vi "getHelpQuestionmark.vi"(8 "error in (no error)":errorcluster, 11 "TEI9150 in":refnum<class "TEI9150.lvclass">) -> (0 "error out":errorcluster, 2 "Items and Unit Numbers":string, 3 "TEI9150 out":refnum<class "TEI9150.lvclass">)   [LabVIEW 2015, in "TEI9150.lvclass"]
uses:
  TEI9150.lvclass
  TEI9150.lvclass/TEI9150.ctl
  <userlib>/Common/SerialProtocols/SerialCommunicator/SerialCommunicator.lvclass
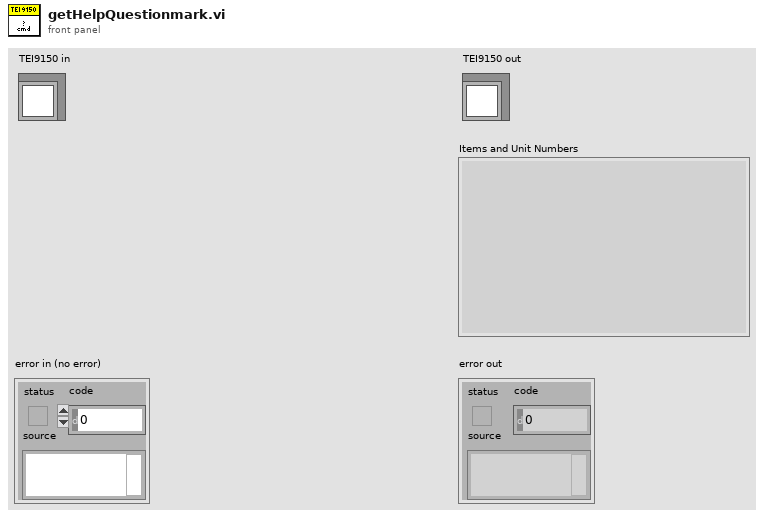
[diagram p1: front panel]
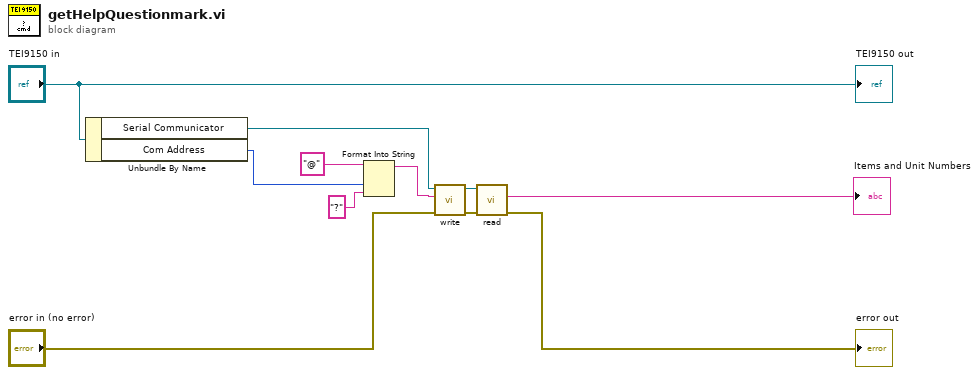
[diagram p0: block diagram]
diagram:
  n1 = Unbundle By Name("TEI9150 in") -> ("Serial Communicator"=w9:refnum<class "SerialCommunicator.lvclass">, "Com Address"=w7:u8)
  n2 = Format Into String(initial string="@", w7, "?" ("input 2")) -> (resulting string=w5:string)  [unwired: 2 in, 1 out]
  n3 = call-dynamic "write.vi"("error in (no error)"="error in (no error)", "writeString"=w5, "SerialCommunicator in"=w9) -> ("error out"=w11:errorcluster, "SerialCommunicator out"=w2:refnum<class "SerialCommunicator.lvclass">)  [unwired: 7 in]
  n4 = call-dynamic "read.vi"("error in (no error)"=w11, "SerialCommunicator in"=w2) -> ("error out"=→"error out":errorcluster, "stringRead"=→"Items and Unit Numbers":string)  [unwired: 7 in, 1 out]
  "TEI9150 out" <- "TEI9150 in"
